vi "Draw Attitude Picture.vi"(7 "draw options":T2={"Text Color"=16777238, "Wing Color"=16751616, "Dial Outline Color"=13816530, "Sky Color"=3381759, "Ground Color"=8213043, "Horizon Line Color"=16777225, "Outline Color"=0, "Dial Background Color"=5987163, "Draw Wings"=TRUE, "Draw Text"=TRUE, "Font Name"="Helvetica", "Angle units"=enum."Degrees"}, 8 "error in (no error)":errorcluster, 9 "DrawAreaSize":T1={"Width"=100, "Height"=100}, 10 "attitude":T4, 11 "picture in":picture) -> (0 "error out":errorcluster, 3 "picture out":picture)   [LabVIEW 2017, in "NI_Robotics_Attitude Picture.lvlib"]
uses:
  <vilib>/robotics/Controls/Attitude Indicator/Attitude Picture/NI_Robotics_Attitude Picture.lvlib
  <vilib>/robotics/Controls/Attitude Indicator/Attitude Picture/Attitude.ctl
  <vilib>/robotics/Controls/Attitude Indicator/Attitude Picture/Draw Options.ctl
  <vilib>/robotics/Controls/Utilities/Angle Units.ctl
  <vilib>/Utility/miscctls.llb/LVBoundsTypeDef.ctl
  <vilib>/robotics/Controls/Attitude Indicator/Attitude Picture/Draw Ground.vi
  <vilib>/robotics/Controls/Attitude Indicator/Attitude Picture/Draw Horizon.vi
  <vilib>/robotics/Controls/Utilities/Random Unused Color.vi
  <vilib>/robotics/Controls/Attitude Indicator/Attitude Picture/XY to Rotated Pixel Points.vi
  <vilib>/robotics/Controls/Attitude Indicator/Attitude Picture/Build Attitude Text.vi
  <vilib>/robotics/Controls/Utilities/Fit Font Size to Box.vi
  <vilib>/Analysis/coordinate.llb/Wrap Angle.vi
  <vilib>/Analysis/coordinate.llb/Wrap Angle (scalar).vi
  <vilib>/Analysis/coordinate.llb/2D Cartesian Coordinate Rotation.vi
  <vilib>/Analysis/coordinate.llb/2D Cartesian Coordinate Rotation (Array).vi
  <vilib>/picture/picture.llb/Draw Flattened Pixmap.vi
  <vilib>/picture/pictutil.llb/Create Mask.vi
  <vilib>/picture/pictutil.llb/Picture to Pixmap.vi
  <vilib>/picture/pictutil.llb/Draw Circle by Radius.vi
  <vilib>/picture/picture.llb/Draw Text at Point.vi
  <vilib>/picture/picture.llb/Draw Rect.vi
  <vilib>/picture/picture.llb/Get Text Rect.vi
  <vilib>/Utility/AngleManip/Radians to Degrees.vi
  <vilib>/Utility/AngleManip/Radians to Degrees (Scalar DBL).vi
  <vilib>/picture/picture.llb/Draw Multiple Lines.vi
  <vilib>/picture/picture.llb/Draw Point.vi
  <vilib>/Utility/AngleManip/Degrees to Radians.vi
  <vilib>/Utility/AngleManip/Degrees to Radians (Scalar DBL).vi
  <vilib>/Utility/AngleManip/Degrees to Radians (Array DBL).vi
  <vilib>/robotics/Controls/Utilities/NI_Robotics_Control Utilities.lvlib
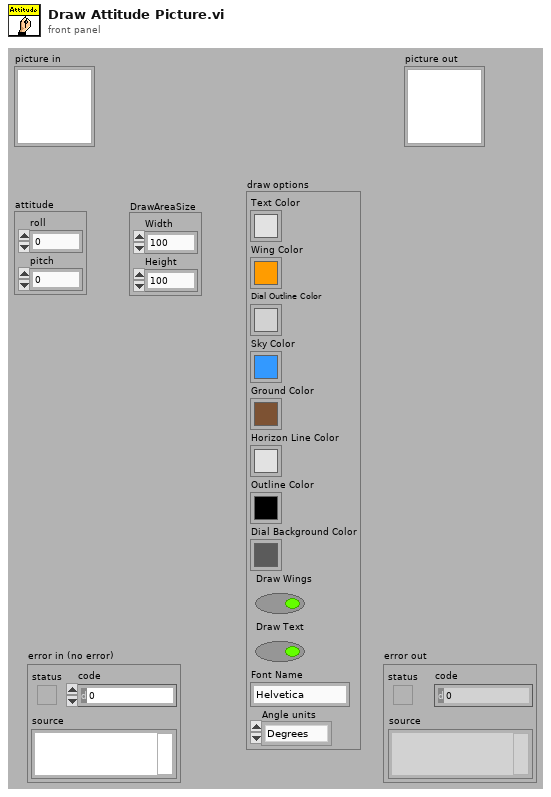
[diagram p1: front panel]
types:
  T1 = typedef "LVBoundsTypeDef.ctl" = cluster{"Width":u32, "Height":u32}
  T2 = typedef "NI_Robotics_Attitude Picture.lvlib/Draw Options.ctl" = cluster{"Text Color":u32, "Wing Color":u32, "Dial Outline Color":u32, "Sky Color":u32, "Ground Color":u32, "Horizon Line Color":u32, "Outline Color":u32, "Dial Background Color":u32, "Draw Wings":bool, "Draw Text":bool, "Font Name":string, "Angle units":T3}
  T3 = typedef "NI_Robotics_Control Utilities.lvlib/Angle Units.ctl" = enum16{"Radians", "Degrees"}
  T4 = typedef "NI_Robotics_Attitude Picture.lvlib/Attitude.ctl" = cluster{"roll":dbl, "pitch":dbl}
  T5 = typedef "NI_Robotics_Attitude Picture.lvlib/Draw Area State.ctl" = cluster{"center":cluster{"x":i16, "y":i16}, "Thick Pen":cluster{"Width":u16, "Style":enum32{"Solid", "Dash", "Dot", "DashDot", "DashDotDot"}}, "Medium Pen":cluster{"Width":u16, "Style":enum32{"Solid", "Dash", "Dot", "DashDot", "DashDotDot"}}, "DrawAreaSize":T1, "pixels per unit":dbl, "units per radian":dbl}
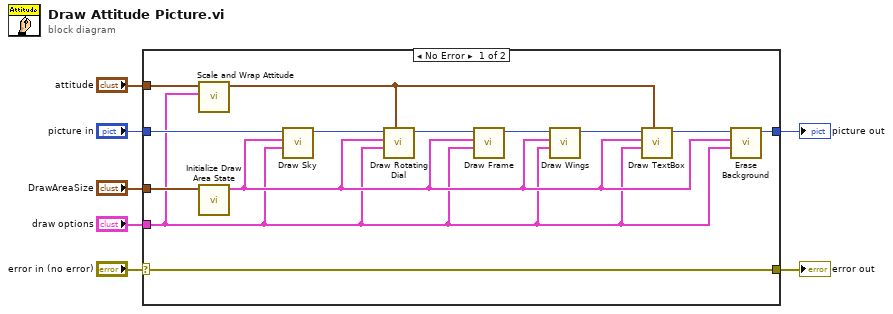
[diagram p0: block diagram]
diagram:
  n1 = case shown="No Error" "error in (no error)" {
    selector: "error in (no error)" -> [w8 w21]
    tunnel: [w20 w22] -> w7
    tunnel: "DrawAreaSize" -> [w15 _]
    tunnel: "picture in" -> [w14 w22]
    tunnel: "attitude" -> [w10 _]
    tunnel: "draw options" -> [w9 _]
    tunnel: [w8 w21] -> w1
    frame No Error {
      n2 = call <vilib>:"Scale and Wrap Attitude.vi"("draw options"=w9, "attitude"=w10) -> ("attitude (rad)"=w11:T4)  [unwired: 9 in]
      n3 = call <vilib>:"Initialize Draw Area State.vi"("DrawAreaSize"=w15) -> ("draw area state"=w12:T5)  [unwired: 10 in]
      n4 = call <vilib>:"Draw Sky.vi"("draw options"=w9, "draw area state"=w12, "picture in"=w14) -> ("picture out"=w13:picture)  [unwired: 8 in]
      n5 = call <vilib>:"Draw Rotating Dial.vi"("attitude (rad)"=w11, "draw options"=w9, "draw area state"=w12, "picture in"=w13) -> ("picture out"=w19:picture)  [unwired: 7 in]
      n6 = call <vilib>:"Draw Frame.vi"("draw options"=w9, "draw area state"=w12, "picture in"=w19) -> ("picture out"=w18:picture)  [unwired: 8 in]
      n7 = call <vilib>:"Draw Wings.vi"("draw options"=w9, "draw area state"=w12, "picture in"=w18) -> ("picture out"=w17:picture)  [unwired: 8 in]
      n8 = call <vilib>:"Draw TextBox.vi"("attitude (rad)"=w11, "draw options"=w9, "draw area state"=w12, "picture in"=w17) -> ("picture out"=w16:picture)  [unwired: 7 in]
      n9 = call <vilib>:"Erase Background.vi"("draw options"=w9, "draw area state in"=w12, "picture in"=w16) -> ("picture out"=w20:picture)  [unwired: 8 in]
    }
    frame Error {
    }
  }
  "picture out" <- w7
  "error out" <- w1
